vi "ValChange.vi"(11 "Data":variant) -> (3 "ValChange":bool)   [LabVIEW 2018]
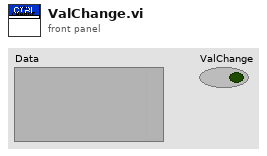
[diagram p1: front panel]
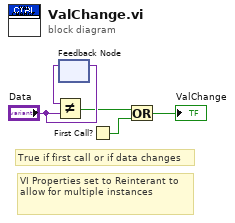
[diagram p0: block diagram]
diagram:
  # "VI Properties set to Reinterant to allow for multiple instances"
  # "True if first call or if data changes"
  n1 = feedback #1() -> (w4:variant)  [unwired: 1 in]
  n2 = Not Equal?(x=w4, y="Data") -> (x != y?=w3:bool)
  n3 = feedback-in #1("Data") -> ()
  n4 = First Call?() -> (First Call?: T/F=w2:bool)
  n5 = Or(x=w3, y=w2) -> (x .or. y?=→"ValChange":bool)
